vi "start.vi"(6 "h":i32, 7 "w":i32, 8 "error in (no error)":errorcluster, 9 "Mbuf":refnum<k24>, 10 "new reference in":refnum<k24>, 11 ".NET Refnum in":refnum<k24>) -> (0 "error out":errorcluster, 1 "buf out":u16[][](array[numeric]), 3 ".NET Refnum out":refnum<k24>)   [LabVIEW 2019]
uses:
  C:/Users/huang/Desktop/MIL LITE 10/64/Matrox Imaging/MIL/MIL.NET/Matrox.MatroxImagingLibrary.v3.5.dll
  64/Matrox Imaging/MIL/MIL.NET/Matrox.MatroxImagingLibrary.v3.5.dll
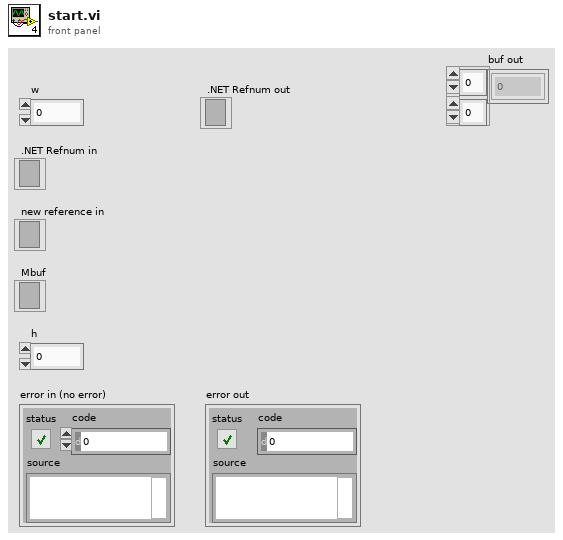
[diagram p1: front panel]
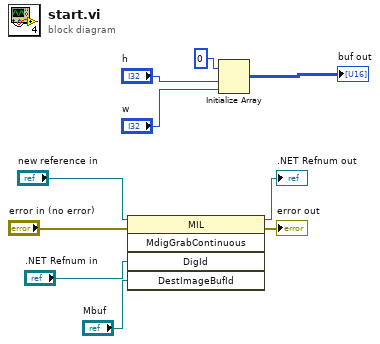
[diagram p0: block diagram]
diagram:
  n1 = invoke on="调用节点" class="MIL" method="MdigGrabContinuous"(reference="new reference in", error in="error in (no error)", "DigId"=".NET Refnum in", "DestImageBufId"="Mbuf") -> (reference out=→".NET Refnum out":refnum<k24>, error out=→"error out":errorcluster)  [unwired: 1 in, 3 out]
  n2 = Initialize Array(u16 0 ("element"), "h", "w") -> (→"buf out":u16[][])
